vi "Construct.vi"(8 "error in (no error)":errorcluster, 9 "Resource Data ref":refnum<data-value>, 10 "Project Path":path=path "") -> (0 "error out":errorcluster, 3 "Project Data out":refnum<class "Project Data.lvclass">)   [LabVIEW 2013, in "SET Project Data.lvlib" / "Project Data.lvclass"]
uses:
  Project Data.lvclass
  Resource Data Class/Resource Data.lvclass
  Project Data.lvclass/Project Data.ctl
  SET Project Data.lvlib
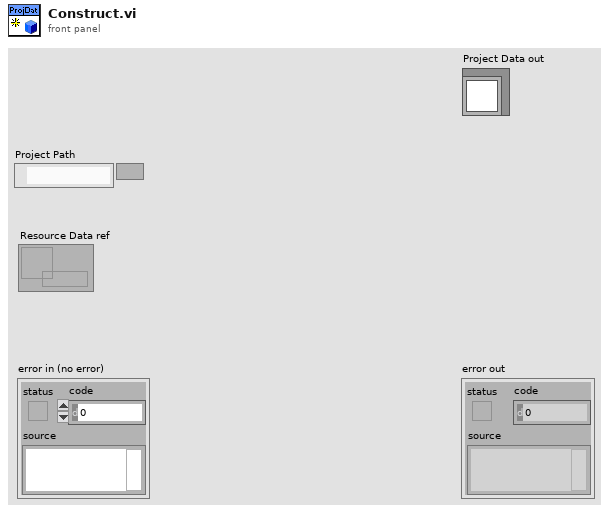
[diagram p1: front panel]
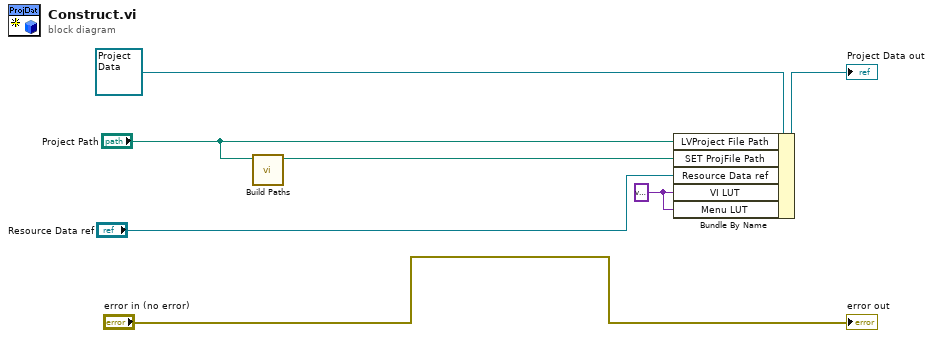
[diagram p0: block diagram]
diagram:
  w3 = variant ("VI LUT")
  n1 = call "Build Paths.vi"("lvproj Path"="Project Path") -> ("SET ProjFile Path"=w4:path)  [unwired: 10 in]
  n2 = Bundle By Name(cluster=refnum<class "Project Data.lvclass"> refnum ("LanguageData in"), "LVProject File Path"="Project Path", "SET ProjFile Path"=w4, "Resource Data ref"="Resource Data ref", "VI LUT"=w3, "Menu LUT"=w3) -> (→"Project Data out":refnum<class "Project Data.lvclass">)
  "error out" <- "error in (no error)"
